vi "Buffer Storage Status.vi"(8 "error in (no error)":errorcluster, 11 "VISA resource name":refnum<visa-resource-name>) -> (0 "error out":errorcluster, 1 "Number of Stored Readings":string, 2 "Points Remaining":string, 3 "VISA resource name out":refnum<visa-resource-name>, 4 "Operation Complete?":bool)   [LabVIEW 2018, in "BK Precision 8600 Series.lvlib"]
doc: "Checks the current status of the buffer storage operation. It returns the number of points (readings) to measure and store into the buffer and the number of readings already stored into the buffer."
uses:
  <instrlib>/BK Precision 8600 Series/BK Precision 8600 Series.lvlib
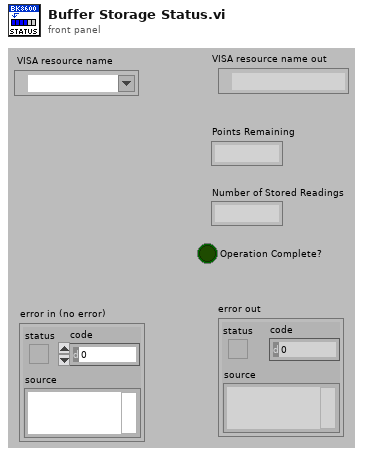
[diagram p1: front panel]
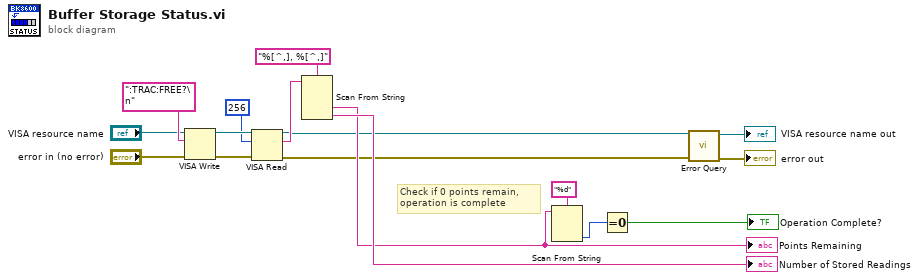
[diagram p0: block diagram]
diagram:
  # "Check if 0 points remain,\noperation is complete"
  n1 = VISA Write(VISA resource name="VISA resource name", write buffer=":TRAC:FREE?\n", error in (no error)="error in (no error)") -> (VISA resource name out=w13:refnum<visa-resource-name>, error out=w14:errorcluster)  [unwired: 1 out]
  n2 = VISA Read(VISA resource name=w13, byte count=256, error in (no error)=w14) -> (VISA resource name out=w4:refnum<visa-resource-name>, read buffer=w11:string, error out=w3:errorcluster)  [unwired: 1 out]
  n3 = Scan From String(format string="%[^,], %[^,]", input string=w11) -> (output 1=w6:string, output 2=→"Number of Stored Readings":string)  [unwired: 4 in, 3 out]
  "Points Remaining" <- w6
  n4 = Scan From String(format string="%d", input string=w6) -> (output 1=w5:i32)  [unwired: 3 in, 3 out]
  n5 = Equal To 0?(x=w5) -> (x = 0?=→"Operation Complete?":bool)
  n6 = call <instrlib>:"Error Query.vi"("error in (no error)"=w3, "VISA resource name"=w4) -> ("error out"=→"error out":errorcluster, "VISA resource name out"=→"VISA resource name out":refnum<visa-resource-name>)  [unwired: 6 in, 2 out]
